vi "InitializeNextron.vi"(8 "error in (no error)":errorcluster, 11 "VISA Refnum in":refnum<visa-resource-name>) -> (0 "error in (no error) 2":errorcluster, 2 "read buffer":string, 3 "VISA Refnum Out":refnum<visa-resource-name>)   [LabVIEW 2023]
uses:
  <vilib>/Instr/_visa.llb/VISA Configure Serial Port (Instr).vi
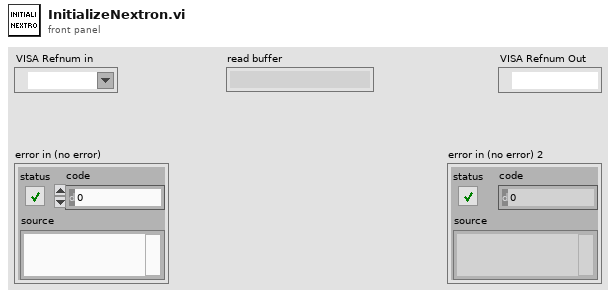
[diagram p1: front panel]
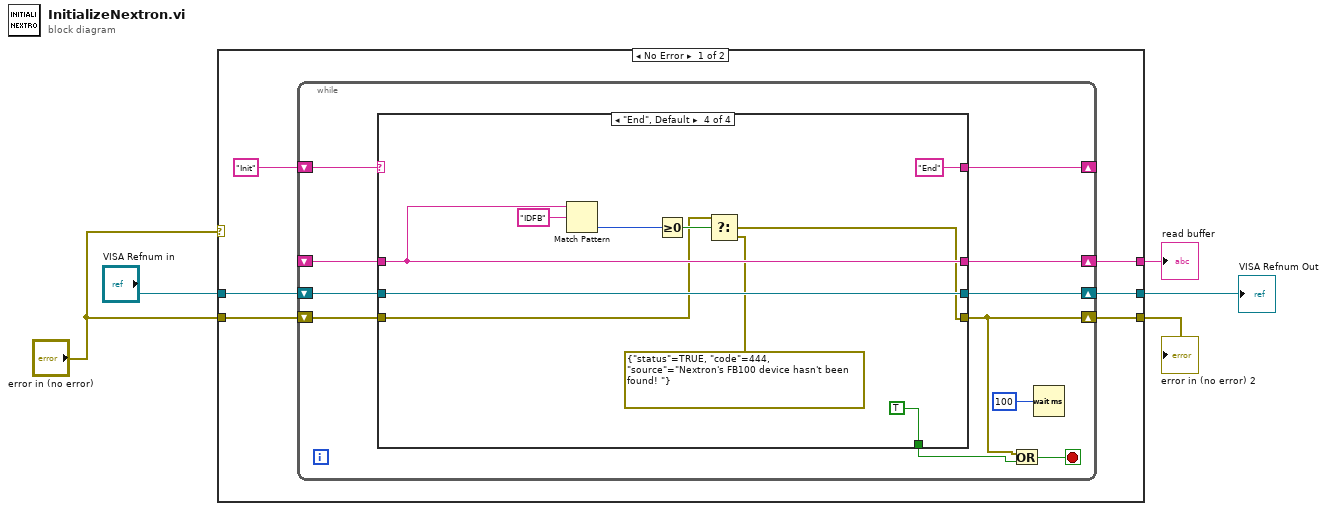
[diagram p0: block diagram]
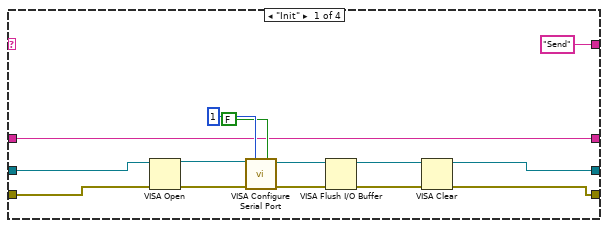
[diagram p2: hidden frame]
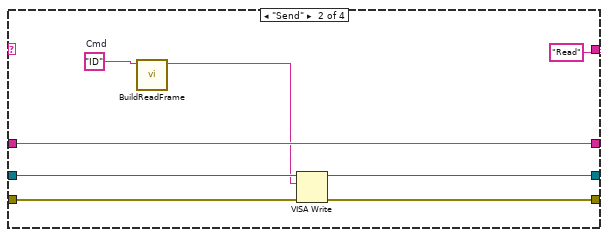
[diagram p3: hidden frame]
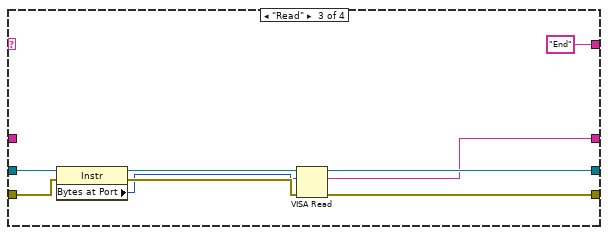
[diagram p4: hidden frame]
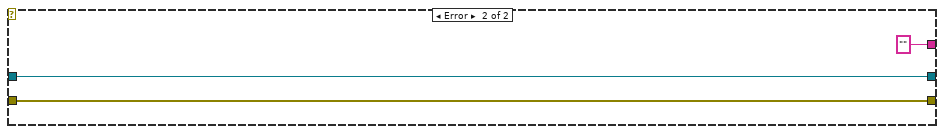
[diagram p5: hidden frame]
diagram:
  n1 = case shown="No Error" "error in (no error)" {
    tunnel: "VISA Refnum in" -> [w11 w65]
    tunnel: "error in (no error)" -> [w10 w64]
    tunnel: [w8 "" ("read buffer")] -> w3
    tunnel: [w7 w65] -> w1
    tunnel: [w6 w64] -> w2
    frame No Error {
      n2 = while {
        shift-right: [w19] -> _
        shift-left: "Init" -> [w20]
        shift-right: [w14] -> w7
        shift-left: w11 -> [w22]
        shift-right: [w15] -> w6
        shift-left: w10 -> [w21]
        shift-right: [w13] -> w8
        shift-left: _ -> [w12]
        stop <- w17 stop-if-true
        n3 = case shown="\"End\", Default" w20 {
          tunnel: w22 -> [w35 w43 w53 w62]
          tunnel: w21 -> [w34 w42 w52 w56]
          tunnel: ["Send" "Read" "End" "End"] -> w19
          tunnel: [_ _ _ TRUE] -> w16
          tunnel: [w24 w40 w47 w55] -> w15
          tunnel: [w25 w39 w48 w62] -> w14
          tunnel: [w23 w38 w46 w60] -> w13
          tunnel: w12 -> [w23 w38 _ w60]
          frame "Init" {
            n4 = VISA Open(error in (no error)=w34, VISA resource name=w35) -> (VISA resource name=w33:refnum<visa-resource-name>, error out=w32:errorcluster)  [unwired: 3 in]
            n5 = call-poly "VISA Configure Serial Port"("VISA resource name"=w33, "timeout (10sec)"=u32 1, "Enable Termination\nChar (T)"=FALSE ("Enable Termination\nChar (T)"), "error in (no error)"=w32) -> ("VISA resource name out"=w29:refnum<visa-resource-name>, "error out"=w28:errorcluster)  [unwired: 10 in]
            n6 = VISA Flush I/O Buffer(VISA resource name=w29, error in (no error)=w28) -> (VISA resource name out=w27:refnum<visa-resource-name>, error out=w26:errorcluster)  [unwired: 1 in]
            n7 = VISA Clear(VISA resource name=w27, error in (no error)=w26) -> (VISA resource name out=w25:refnum<visa-resource-name>, error out=w24:errorcluster)
          }
          frame "Send" {
            w44 = "ID"  # Cmd
            n8 = call "BuildReadFrame.vi"("Cmd"=w44) -> ("String"=w37:string)  [unwired: 10 in]
            n9 = VISA Write(VISA resource name=w43, write buffer=w37, error in (no error)=w42) -> (VISA resource name out=w39:refnum<visa-resource-name>, error out=w40:errorcluster)  [unwired: 1 out]
          }
          frame "Read" {
            n10 = property class="Instr"(reference=w53, error in=w52) -> (reference out=w51:refnum<visa-resource-name>, error out=w50:errorcluster, "Bytes at Port"=w49:u32)
            n11 = VISA Read(VISA resource name=w51, byte count=w49, error in (no error)=w50) -> (VISA resource name out=w48:refnum<visa-resource-name>, read buffer=w46:string, error out=w47:errorcluster)  [unwired: 1 out]
          }
          frame "End", Default {
            n12 = Match Pattern(string=w60, regular expression="IDFB") -> (offset past match=w58:i32)  [unwired: 1 in, 3 out]
            n13 = Greater Or Equal To 0?(x=w58) -> (x >= 0?=w57:bool)
            n14 = Select(t=w56, s=w57, f=errorcluster {"status"=TRUE, "code"=444, "source"="Nextron's FB100 device hasn't been found! "}) -> (s? t:f=w55:errorcluster)
          }
        }
        n15 = Or(x=w15, y=w16) -> (x .or. y?=w17:bool)
        n16 = Wait (ms)(milliseconds to wait=u32 100) -> ()  [unwired: 1 out]
      }
    }
    frame Error {
    }
  }
  "read buffer" <- w3
  "VISA Refnum Out" <- w1
  "error in (no error) 2" <- w2
